vi "StopListener.vi"(0 "reference":refnum<class "VdTcpIP.lvclass">, 5 "error in (no error)":errorcluster) -> (14 "reference out":refnum<class "VdTcpIP.lvclass">, 19 "error out":errorcluster)   [LabVIEW 2020, in "VdTcpIP.lvclass"]
doc: "Stops the listener process"
uses:
  VdTcpIP.lvclass
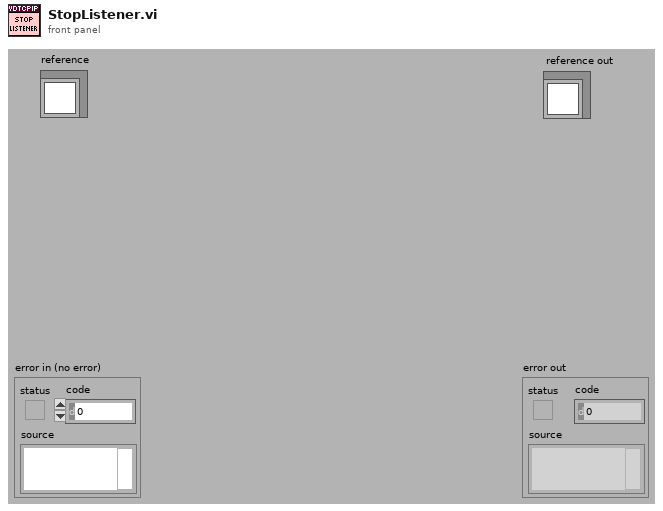
[diagram p1: front panel]
types:
  T1 = typedef "VdTcpIP.lvclass/ObjectAttributes.ctl" = cluster{"IP-Address":string, "Port":u16, "Connection":refnum<k5>, "Listener":refnum<k5>, "ListenerConnection":refnum<k5>, "Listner":bool, "ListnerProcessRunning":bool, "InConnections":refnum<k5>[], "InConnectionsIP":string[], "InConnectionAdded":refnum<notifier>, "RunVIOnNewConnection":variant, "DataToNewConnectionVI":cluster{"ControlName":string, "ControlValue":variant}[], "WebServicesURL_Location(http://...)":string, "WebServicesPostWebPage(*.asmx)":string, "Semaphore":T2, "AutoReConnectTimes":i32, "AutoReConnectInterval(ms)":i32, "ConnectionTimeout":i32}
  T2 = typedef "Semaphore RefNum" = refnum<k1>
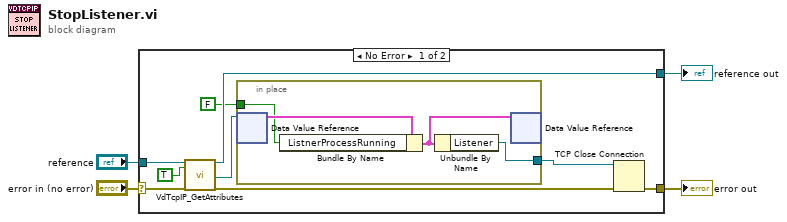
[diagram p0: block diagram]
diagram:
  n1 = case shown="No Error" "error in (no error)" {
    selector: "error in (no error)" -> [w13 w18]
    tunnel: "reference" -> [w12 w19]
    tunnel: [w9 w18] -> w2
    tunnel: [w11 w19] -> w1
    frame No Error {
      n2 = call "VdTcpIP_GetAttributes.vi"("reference in"=w12, "OnlyGetDvrReference(False)"=TRUE, "error in (no error)"=w13) -> ("reference out"=w11:refnum<class "VdTcpIP.lvclass">, "DataRef"=w7:refnum<data-value>, "error out"=w10:errorcluster)  [unwired: 13 in, 1 out]
      n3 = in-place {
        in-place-border: FALSE ("ListnerProcessRunning") -> [w16]
        in-place-border: [w15] -> w5
        n4 = in-place-dvr #1(w7) -> (w17:T1)  [unwired: 1 out]
        n5 = Bundle By Name(cluster=w17, "ListnerProcessRunning"=w16) -> (w14:T1)
        n6 = Unbundle By Name(w14) -> ("Listener"=w15:refnum<k5>)
        n7 = in-place-dvr #1(w14) -> ()  [unwired: 2 out]
      }
      n8 = TCP Close Connection(connection ID=w5, error in (no error)=w10) -> (error out=w9:errorcluster)  [unwired: 2 out]
    }
    frame Error {
    }
  }
  "reference out" <- w1
  "error out" <- w2
